vi "Test Screen Size.vi"() -> ()   [LabVIEW 2013]
uses:
  <vilib>/Utility/miscctls.llb/LVRectTypeDef.ctl
panel:
  out "x+y 2":dbl
  out "x+y":dbl
  out "Bounds:Area Width":u32
  out "Front Panel Window:Panel Bounds":T1
  in  "Tab Control":enum32{"Page 1", "Page 2"}(tab)
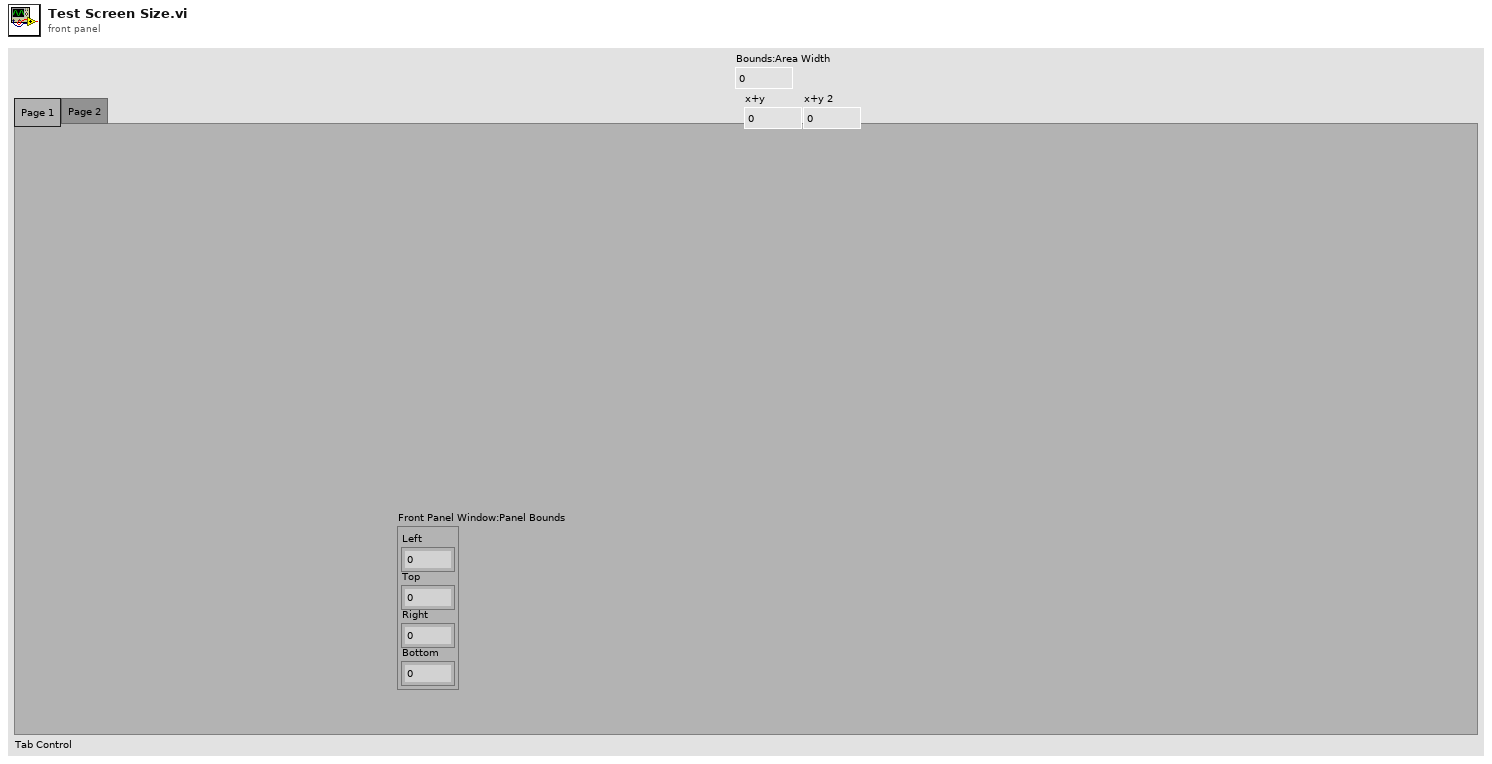
[diagram p1: front panel]
types:
  T1 = typedef "LVRectTypeDef.ctl" = cluster{"Left":i16, "Top":i16, "Right":i16, "Bottom":i16}
  T2 = enum32{"Invalid", "Standard", "Closed", "Hidden", "Minimized", "Maximized"}
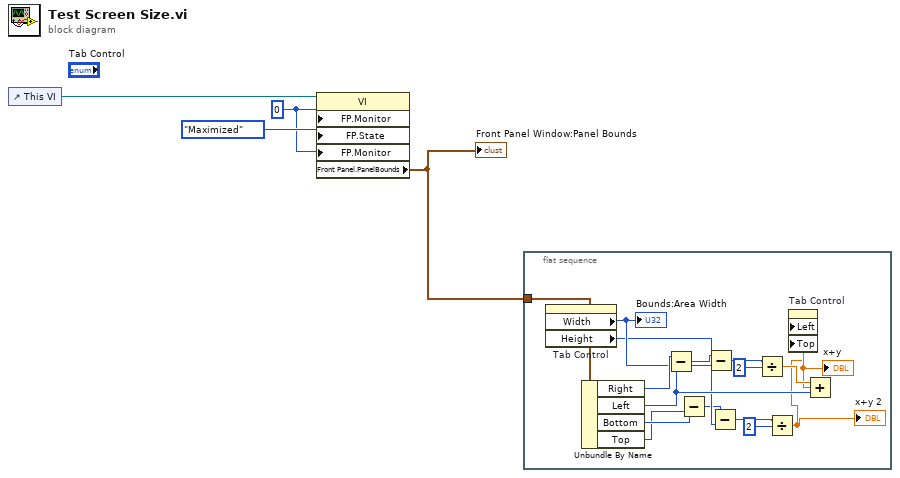
[diagram p0: block diagram]
diagram:
  w2 = u16 0 ("Front Panel Window:Monitor")
  n1 = control-ref of="This VI"() -> (w4:refnum<vi>)
  n2 = property class="VI"(reference=w4, "FP.Monitor"=w2, "FP.State"=T2."Maximized" ("Front Panel Window:State"), "FP.Monitor"=w2) -> ("Front Panel.PanelBounds"=w1:T1)  [unwired: 1 in, 2 out]
  "Front Panel Window:Panel Bounds" <- w1
  n3 = flat-sequence {
    tunnel: w1 -> [w20]
    frame #0 {
      n4 = property on="Tab Control" class="TabCtl (strict)"() -> ("Width"=w17:u32, "Height"=w9:u32)  [unwired: 2 in, 2 out]
      "Bounds:Area Width" <- w17
      n5 = Unbundle By Name(w20) -> ("Right"=w19:i16, "Left"=w12:i16, "Bottom"=w14:i16, "Top"=w6:i16)
      n6 = Subtract(x=w19, y=w12) -> (x-y=w18:i16)
      n7 = Subtract(x=w14, y=w6) -> (x-y=w8:i16)
      n8 = Subtract(x=w18, y=w17) -> (x-y=w16:u32)
      n9 = Subtract(x=w8, y=w9) -> (x-y=w7:u32)
      n10 = Divide(x=w16, y=u32 2) -> (x/y=w13:dbl)
      n11 = Divide(x=w7, y=u32 2) -> (x/y=w5:dbl)
      "x+y 2" <- w5
      n12 = Add(x=w13, y=w12) -> (x+y=w11:dbl)
      "x+y" <- w11
      n13 = property on="Tab Control" class="TabCtl (strict)"("Left"=w11, "Top"=w5) -> ()  [unwired: 2 in, 2 out]
    }
  }
